vi "WPI_CameraGet Image Size.vi"(8 "error in (no error)":errorcluster, 11 "CameraDevRef":T1={"Camera Address"="192.168.0.90", "CameraStatus"={"status"=FALSE, "code"=0, "source"=""}}) -> (0 "error out":errorcluster, 1 "Size W,H (pix)":cluster{i32, i32}, 2 "Image Size":T2, 3 "CameraDevRef Out":T1)   [LabVIEW 2017]
doc: "Returns the size of the image the camera you specify acquired.\n\nThis software is licensed. Open the labview\\readme\\WPI Robotics Library Open Source License.txt file for more information."
uses:
  <vilib>/Rock Robotics/WPI/Camera/WPI_CameraImageSize.ctl
  <vilib>/Rock Robotics/WPI/Camera/WPI_CameraDevRef.ctl
  <vilib>/userdefined/High Color/IMAQdx.ctl
  <resource>/objmgr/imaqdx.rc
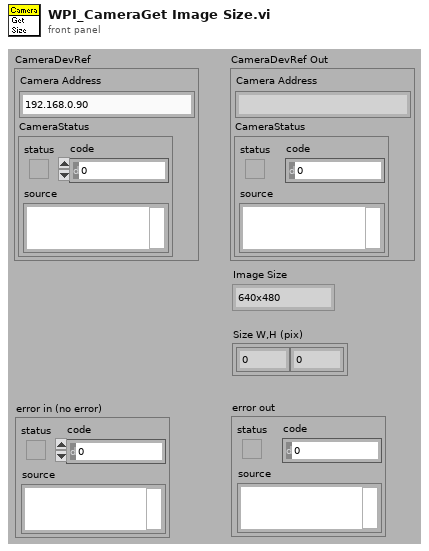
[diagram p1: front panel]
types:
  T1 = typedef "WPI_CameraDevRef.ctl" = cluster{"Camera Address":string, "CameraStatus":errorcluster}
  T2 = typedef "WPI_CameraImageSize.ctl" = enum16{"640x480", "320x240", "160x120", "Custom"}
  T3 = typedef "IMAQdx.ctl" = refnum<k21>
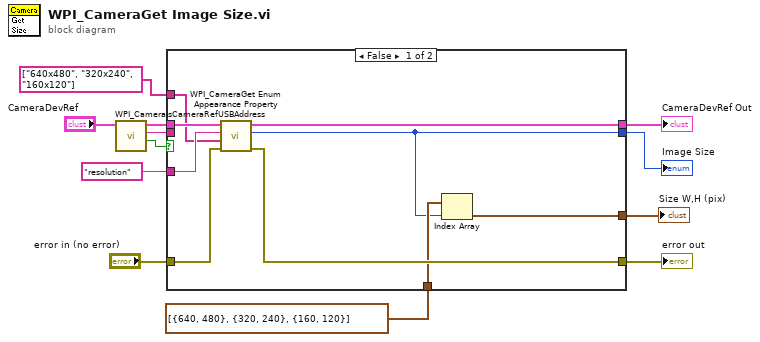
[diagram p0: block diagram]
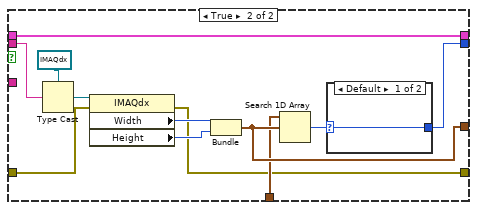
[diagram p2: hidden frame]
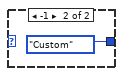
[diagram p3: hidden frame]
diagram:
  n1 = call <vilib>:"WPI_CameraIsCameraRefUSBAddress.vi"("CameraDevRef"="CameraDevRef") -> ("USB?"=w4:bool, "Camera Address Out"=w5:string, "CameraDevRef out"=w2:T1)  [unwired: 7 in, 1 out]
  n2 = case shown="False" w4 {
    tunnel: w2 -> [w21 w33]
    tunnel: "resolution" ("format string") -> [w20 _]
    tunnel: string[] ["640x480", "320x240", "160x120"] -> [w19 _]
    tunnel: "error in (no error)" -> [w18 w23]
    tunnel: [w13 w26] -> w10
    tunnel: [w17 w33] -> w9
    tunnel: [w16 w22] -> w8
    tunnel: w5 -> [_ w32]
    tunnel: [w14 w25] -> w7
    tunnel: cluster{i32, i32}[] [{640, 480}, {320, 240}, {160, 120}] -> [w15 w24]
    frame False {
      n3 = call <vilib>:"WPI_CameraGet Enum Appearance Property.vi"("error in (no error)"=w18, "Strings"=w19, "Property Name"=w20, "CameraDevRef"=w21) -> ("error out"=w16:errorcluster, "Enum Int Value"=w13:i32, "CameraDevRef out"=w17:T1)  [unwired: 5 out]
      n4 = Index Array(array=w15, index=w13) -> (element=w14:cluster{i32, i32})
    }
    frame True {
      n5 = Type Cast(type=T3 refnum ("Session In"), x=w32) -> (*(type *) &x=w30:T3)
      n6 = property class="IMAQdx"(reference=w30, error in=w23) -> (error out=w22:errorcluster, "Width"=w29:u32, "Height"=w28:u32)  [unwired: 1 out]
      n7 = Bundle("Width"=w29, "Height"=w28) -> (w25:cluster{"Width":u32, "Height":u32})  [unwired: 1 in]
      n8 = Search 1D Array(1D array=w24, element=w25) -> (index of element=w27:i32)  [unwired: 1 in]
      n9 = case shown="Default" w27 {
        selector: w27 -> [w34 _]
        tunnel: [w34 WPI_CameraImageSize."Custom" ("Image Size")] -> w26
        frame Default {
        }
        frame -1 {
        }
      }
    }
  }
  "Image Size" <- w10
  "CameraDevRef Out" <- w9
  "error out" <- w8
  "Size W,H (pix)" <- w7
